vi "warten.vi"(8 "error in (no error)":errorcluster caption="Fehler (Eingang, kein Fehler)", 9 "Datenfluss":bool, 11 "Zu wartende ms":u32) -> (0 "error out":errorcluster caption="Fehler (Ausgang)", 3 "Timer-Wert (ms)":u32)   [LabVIEW 2020, in "allgemeine Sub-VIs.lvlib"]
uses:
  allgemeine Sub-VIs.lvlib
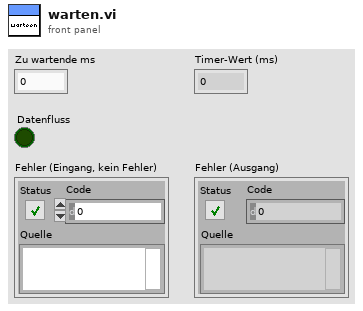
[diagram p1: front panel]
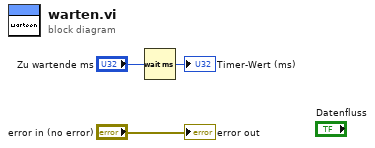
[diagram p0: block diagram]
diagram:
  n1 = Wait (ms)(milliseconds to wait="Zu wartende ms") -> (millisecond timer value=→"Timer-Wert (ms)":u32)
  "error out" <- "error in (no error)"
